vi "Scanner_02.vi"() -> ()   [LabVIEW 2011]
panel:
  out "String":string
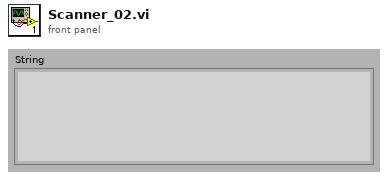
[diagram p1: front panel]
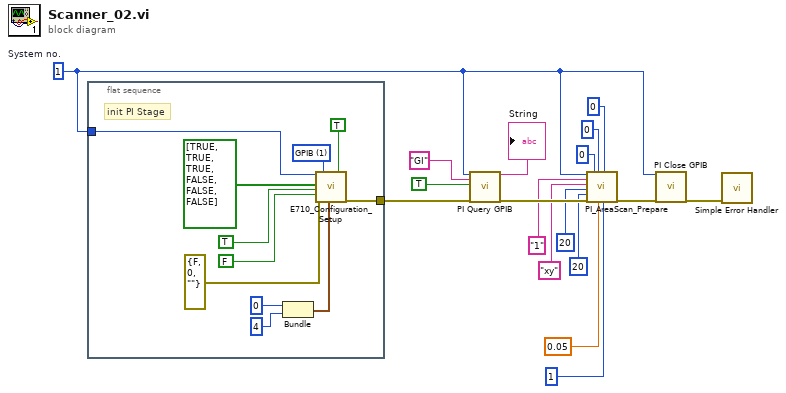
[diagram p0: block diagram]
diagram:
  w11 = 1  # System no.
  n1 = flat-sequence {
    tunnel: [w23] -> w16
    tunnel: w11 -> [w22]
    frame #0 {
      w25 = u16 1 items=["RS232", "GPIB"] ("Interface")
      # "init PI Stage"
      n2 = Bundle(0, 4) -> (w20:cluster{i32, i32})  [unwired: 1 out]
      n3 = call "E710_Configuration_Setup.vi"("System no."=w22, "Are stages connected?"=bool[] [TRUE, TRUE, TRUE, FALSE, FALSE, FALSE], "Change servo \nstatus to ON?"=TRUE ("Change servo \nstatus to ON?"), "Perform autozero?"=FALSE ("All axes?"), "error in"=errorcluster {"status"=FALSE, "code"=0, "source"=""}, "Interface"=w25, "GPIB settings"=w20, "Move to middle?"=TRUE) -> ("error out"=w23:errorcluster)  [unwired: 4 in, 7 out]
    }
  }
  n4 = call "PI Query GPIB.vi"("System no."=w11, "String to send"="GI", "Attach Linefeed?"=TRUE, "error in"=w16) -> ("String read"=→"String":string, "error out"=w12:errorcluster)  [unwired: 13 in, 1 out]
  n5 = call "PI_AreaScan_Prepare.vi"("System"=w11, "Laser"="1", "Axis"="xy", "da"=20, "db"=20, "error in (no error)"=w12, "a0"=0, "b0"=0, "Resolution"=0.05, "c0"=0, "Pixel time"=1) -> ("error out"=w1:errorcluster)  [unwired: 3 in, 5 out]
  n6 = call "PI Close GPIB.vi"("System no."=w11, "error in"=w1) -> ("error out"=w17:errorcluster)  [unwired: 16 in, 1 out]
  n7 = call <vilib>:"Simple Error Handler.vi"("error in (no error)"=w17) -> ()  [unwired: 4 in, 5 out]
